vi "GetCurrentThread (Same As Caller).vi"(8 "error in (no error)":errorcluster, 11 "Impersonate in":refnum<class "LogonUser.lvclass">) -> (0 "error out":errorcluster, 1 "thread id":i64, 3 "Impersonate out":refnum<class "LogonUser.lvclass">)   [LabVIEW 2018, in "LogonUser.lvclass"]
doc: "©2019\nWiebe Walstra\nwww.carya.nl"
uses:
  LogonUser.lvclass
  kernel32.dll
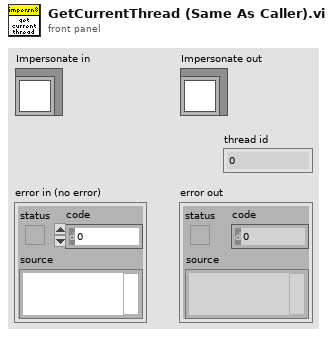
[diagram p1: front panel]
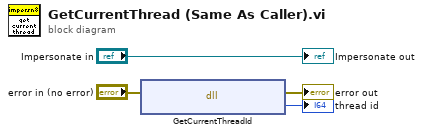
[diagram p0: block diagram]
diagram:
  n1 = dll-call lib="kernel32.dll" fn="GetCurrentThreadId"(error in="error in (no error)") -> (error out=→"error out":errorcluster, "thread"=→"thread id":i64)  [unwired: 2 in, 1 out]
  "Impersonate out" <- "Impersonate in"
